vi "ReadSensorValues_v1.1.vi"(1 "Sample time reference sensor / s":dbl=1.0, 2 "VISA resource name":refnum<visa-resource-name>, 3 "Sensor type":T1) -> ()   [LabVIEW 2012]
uses:
  <vilib>/nican/nicantsk.llb/CAN Interface.ctl
  SensorTypes.ctl
  SensorStates.ctl
  <vilib>/nican/nicantsk.llb/CAN Task Reference.ctl
  <vilib>/nican/nicantsk.llb/CAN Mode.ctl
  globalVariables.vi
  <vilib>/nican/nicantsk.llb/CAN Read Multi Chan Single Samp 1D Dbl.vi
  <instrlib>/Agilent 34970/Agilent 34970.lvlib
panel:
  in  "VISA resource name 2":refnum<visa-resource-name>="USB0::0x0957::0x2007::MY49004365::INSTR"
  in  "Cancel Measurement":bool
  out "new data":bool
  out "running":bool
  out "Sample number":i32
  in  "CAN Interface":T2 items=["CAN0"=0, "CAN1"=1, "CAN2"=2, "CAN3"=3, "CAN4"=4, "CAN5"=5, "CAN6"=6, "CAN7"=7, "CAN8"=8, "CAN9"=9, "CAN10"=10, "CAN11"=11, "CAN12"=12, "CAN13"=13, "CAN14"=14, "CAN15"=15, "CAN16"=16, "CAN17"=17, "CAN18"=18, "CAN19"=19, "CAN20"=20, "CAN21"=21, "CAN22"=22, "CAN23"=23, "CAN24"=24, "CAN25"=25, "CAN26"=26, "CAN27"=27, "CAN28"=28, "CAN29"=29, "CAN30"=30, "CAN31"=31, "CAN32"=32, "CAN33"=33, "CAN34"=34, "CAN35"=35, "CAN36"=36, "CAN37"=37, "CAN38"=38, "CAN39"=39, "CAN40"=40, "CAN41"=41, "CAN42"=42, "CAN43"=43, "CAN44"=44, "CAN45"=45, "CAN46"=46, "CAN47"=47, "CAN48"=48, "CAN49"=49, "CAN50"=50, "CAN51"=51, "CAN52"=52, "CAN53"=53, "CAN54"=54, "CAN55"=55, "CAN56"=56, "CAN57"=57, "CAN58"=58, "CAN59"=59, "CAN60"=60, "CAN61"=61, "CAN62"=62, "CAN63"=63, "MAX default"=64, "CAN256 (Virtual)"=256, "CAN257 (Virtual)"=257]
  out "Error Flag":bool
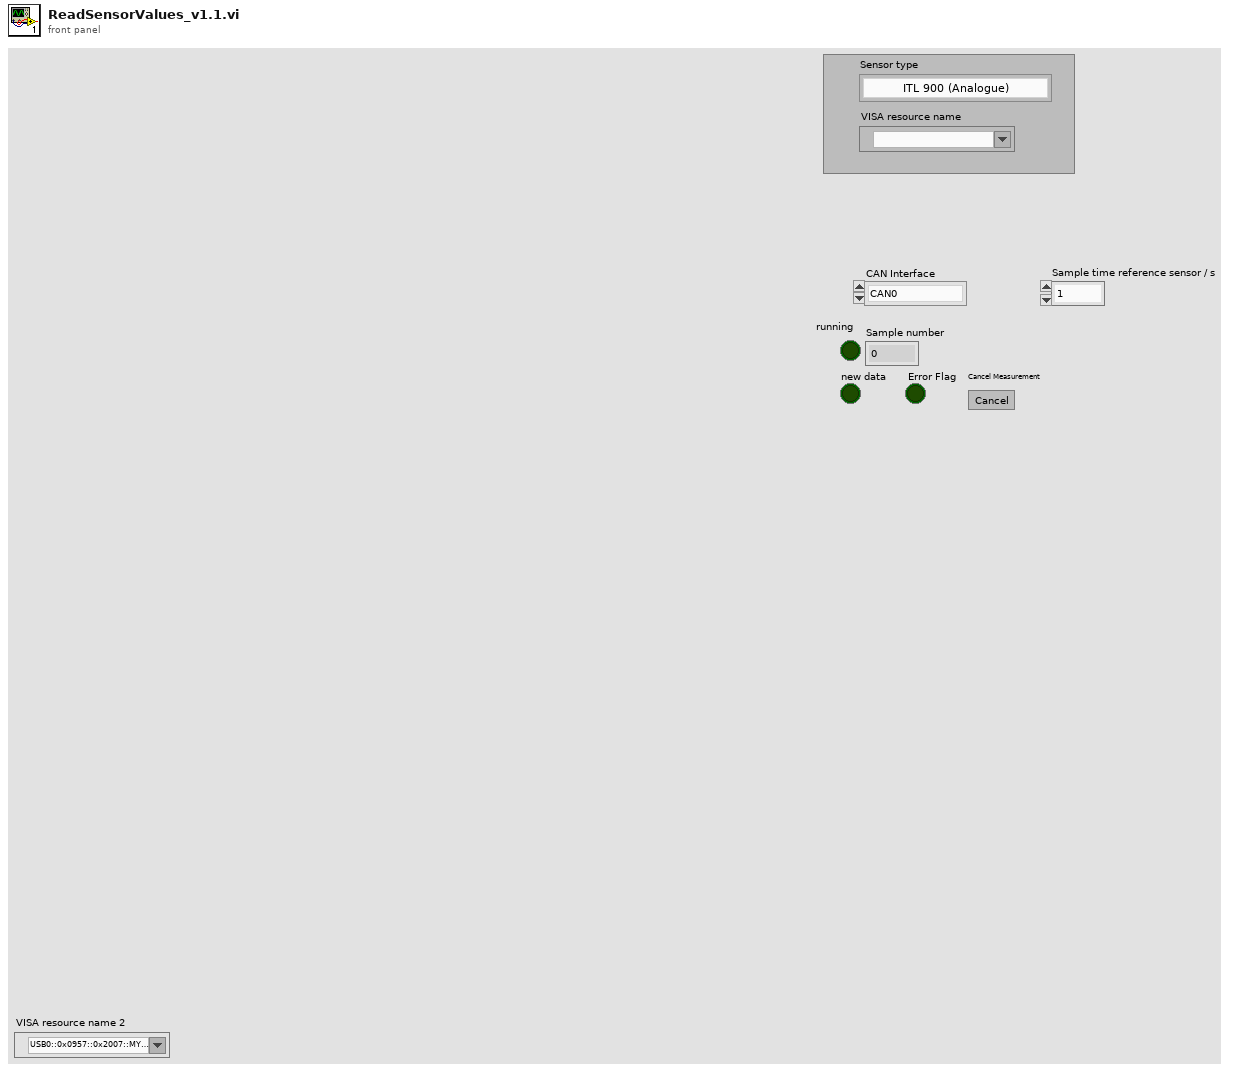
[diagram p1: front panel]
types:
  T1 = typedef "SensorTypes.ctl" = enum16{"ITL 900 (Analogue)", "CAB 300-C SP3 (CAN)", "xyz TODO (PWM)", "xyz TODO (LIN)", "xyz TODO (Analogue)"}
  T2 = typedef "CAN Interface.ctl" = u16
  T3 = typedef "SensorStates.ctl" = enum16{"init", "measure", "terminate"}
  T4 = cluster{"Include Alarm Data F:(No)":bool, "Include Channel # (F:No)":bool, "Include Time (F:No)":bool, "Include Units (F:No)":bool}
  T5 = cluster{"Aperture Value (.4)":dbl, "Aperture (1:Minimum)":u16, "NPLC (1)":u16, "Bandwidth (3 Hz)":u16, "Input Impedance (F:Fixed)":bool, "Integration Time (F:Aperture)":bool}
  T6 = enum16{"100 mV", "1 V", "10 V", "100 V", "300 V", "Minimum", "Maximum"}
  T7 = enum16{"Manual", "Minimum", "Maximum", "Infinity"}
  T8 = enum16{"Bus", "Immediate", "External", "Alarm 1", "Alarm 2", "Alarm 3", "Alarm 4", "Timer"}
  T9 = cluster{"Timeout Value (10000)":u32, "Baud Rate (57600)":enum16{"1200", "2400", "4800", "9600", "19200", "38400", "57600", "115200"}, "Flow Control (1:XON/XOFF)":enum16{"None", "XON / XOFF", "RTS / CTS", "DTR / DSR"}}
  T10 = typedef "CAN Task Reference.ctl" = u32
  T11 = enum16{"Remote Trigger", "Immediate Trigger", "Wait for Trigger", "Abort Scan"}
  T12 = typedef "CAN Mode.ctl" = u16
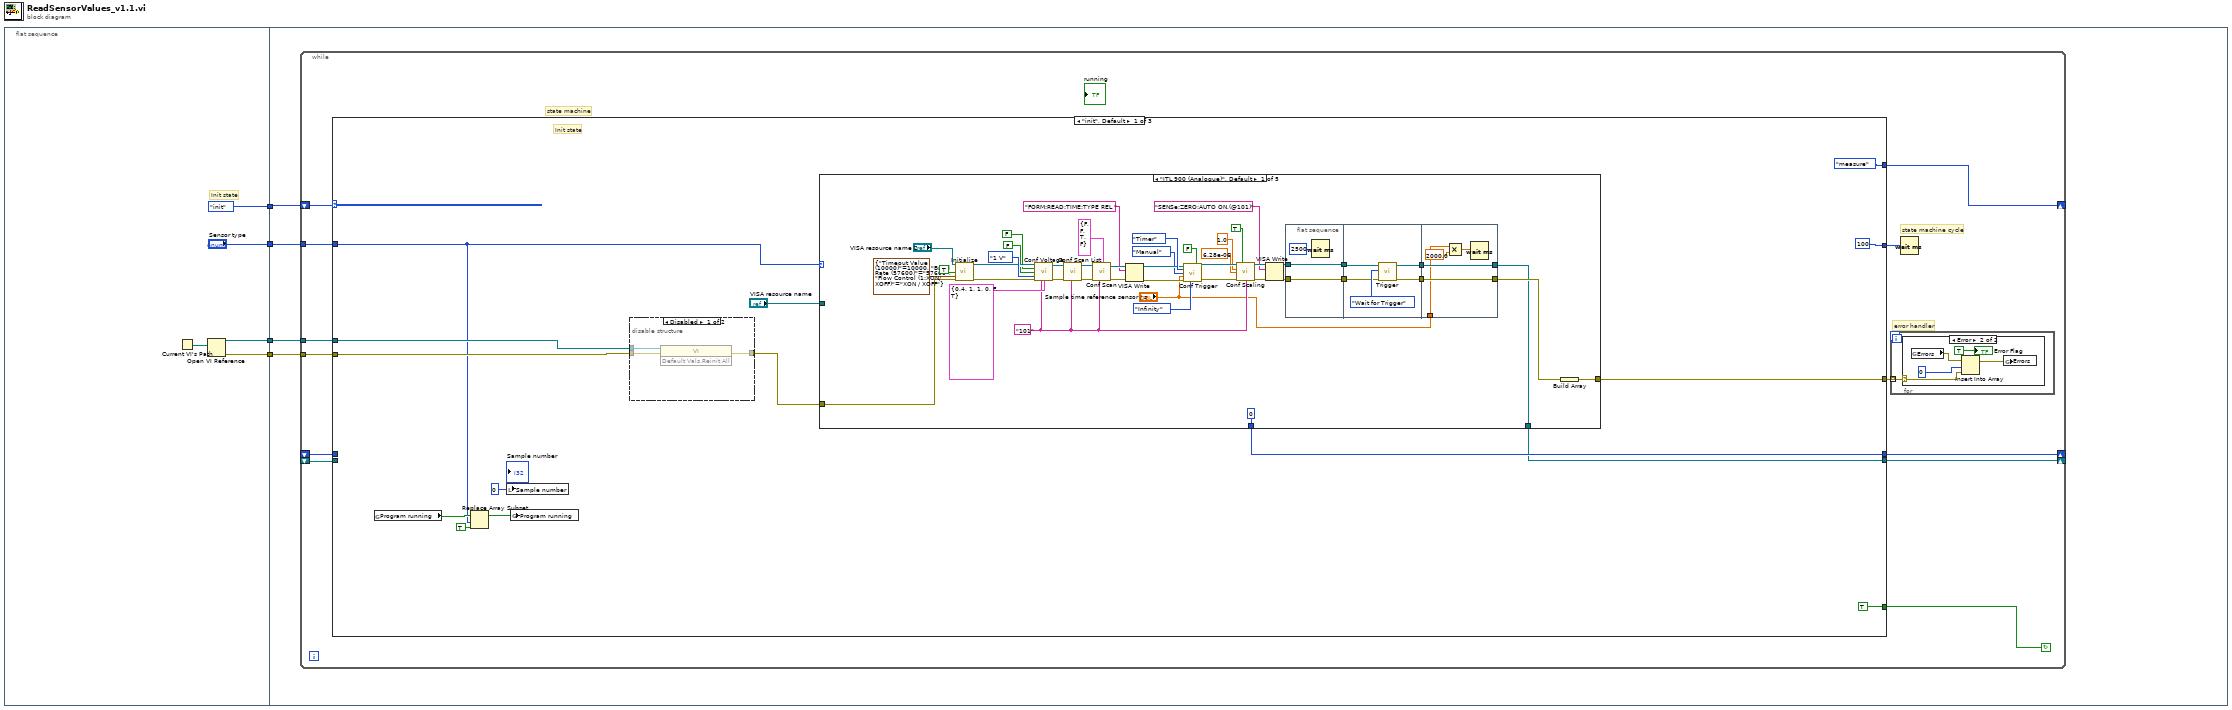
[diagram p0: block diagram]
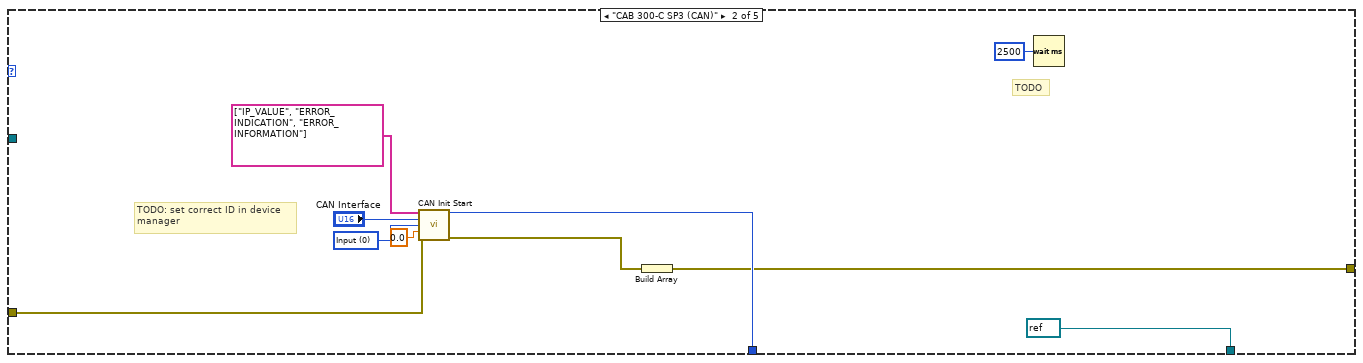
[diagram p4: hidden frame]
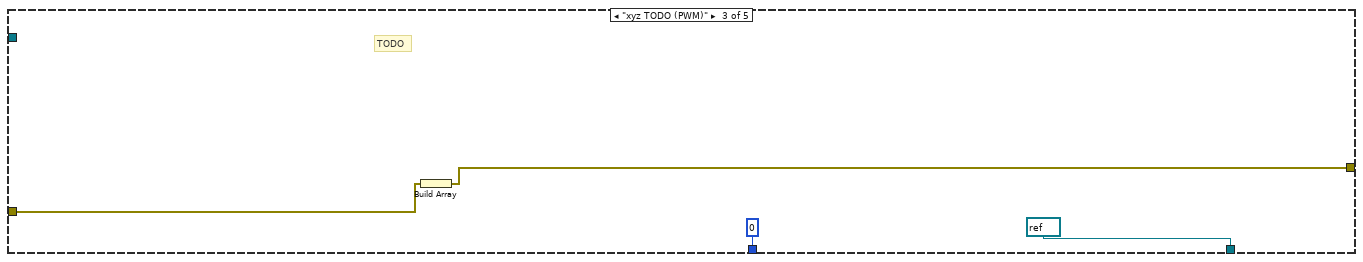
[diagram p5: hidden frame]
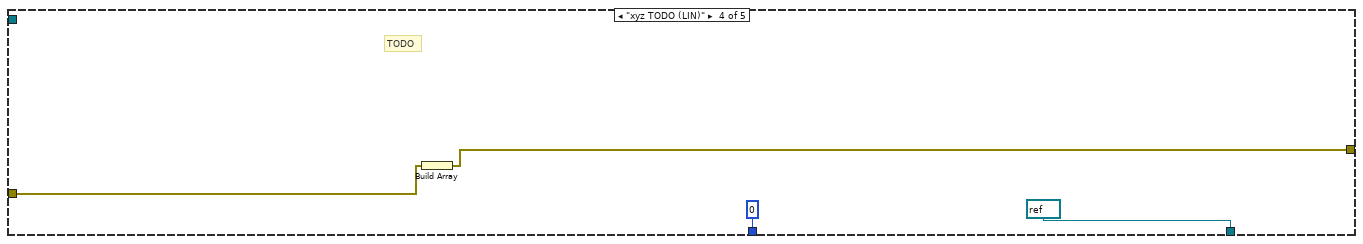
[diagram p6: hidden frame]
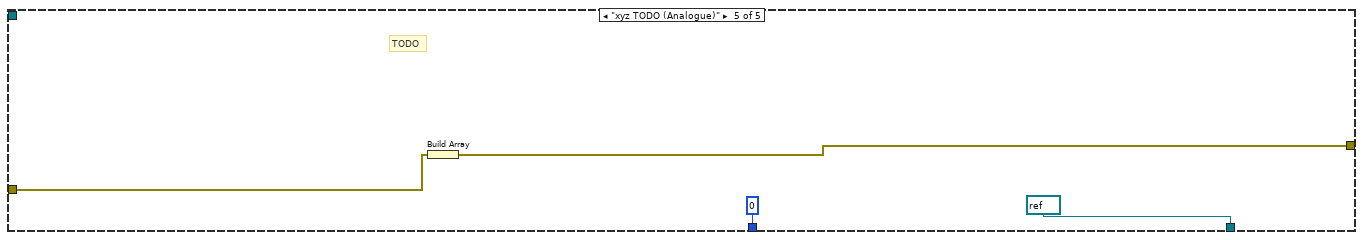
[diagram p7: hidden frame]
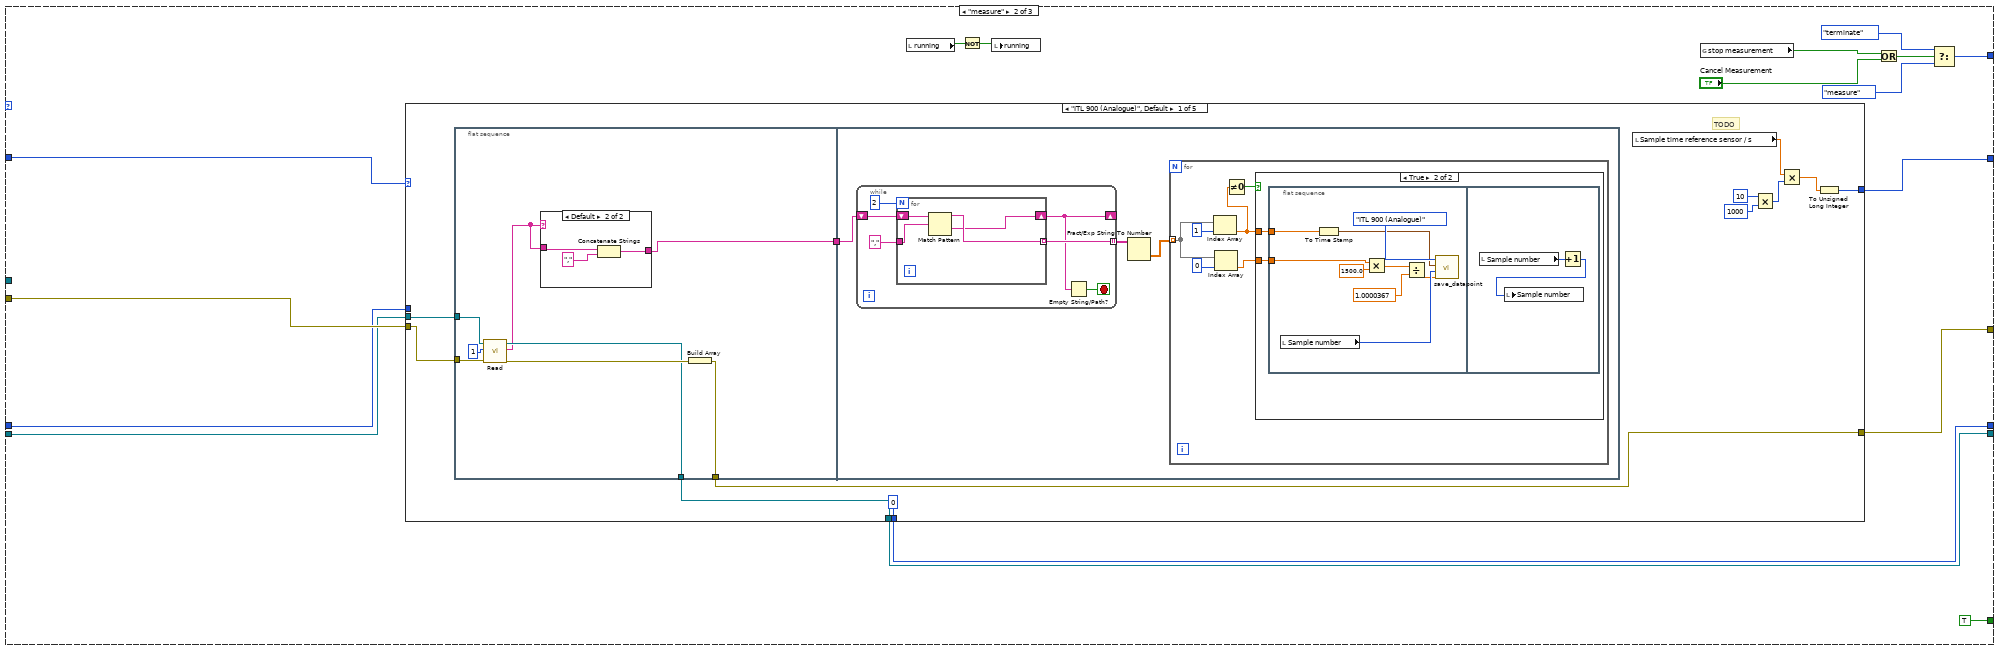
[diagram p8: hidden frame]
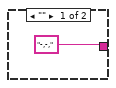
[diagram p9: hidden frame]
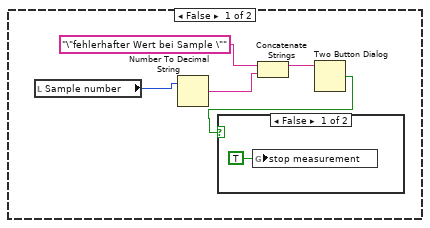
[diagram p10: hidden frame]
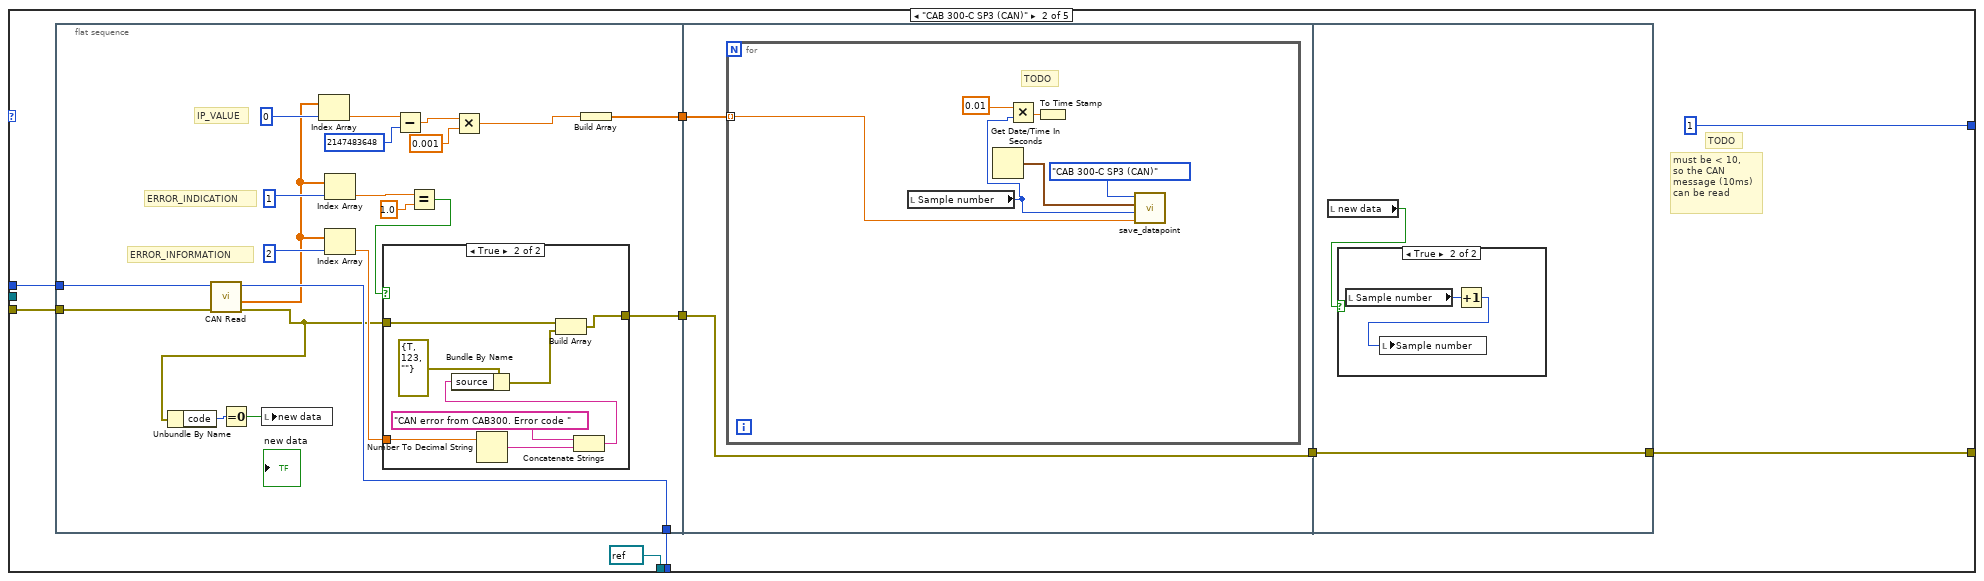
[diagram p12: hidden frame]
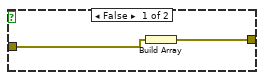
[diagram p13: hidden frame]
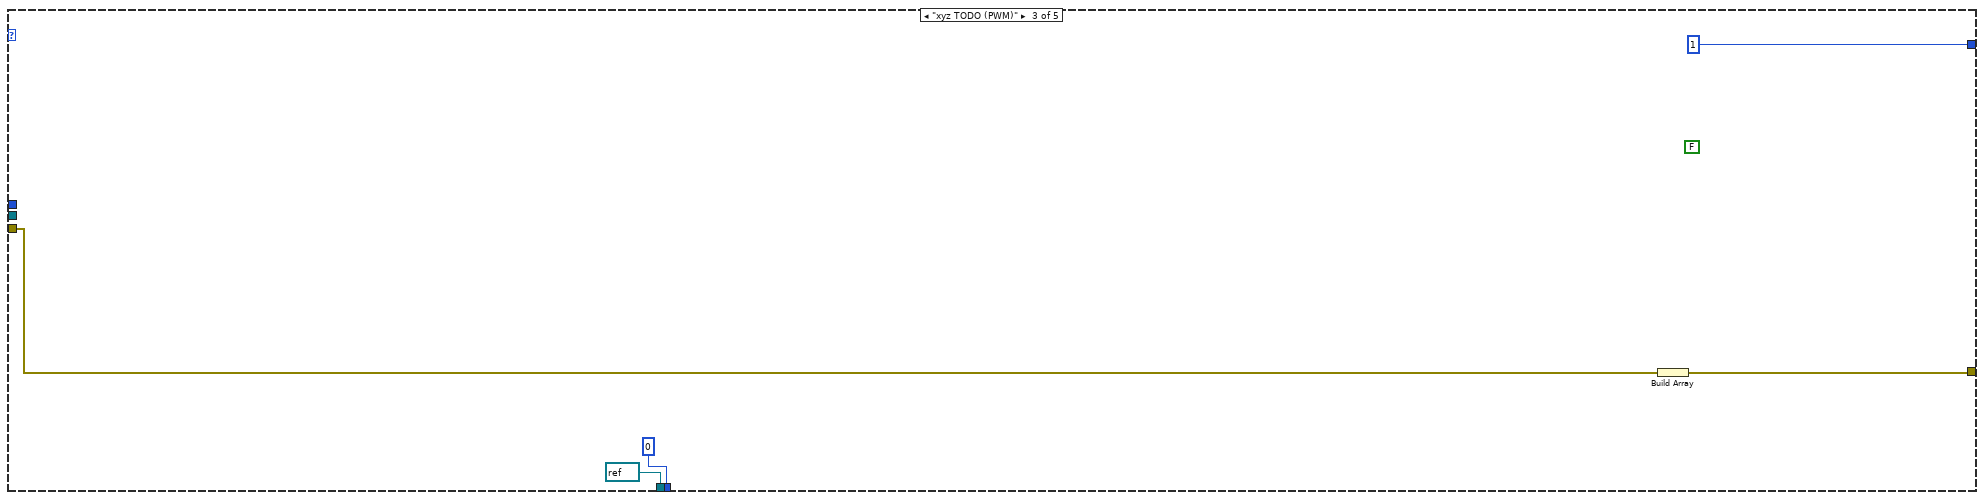
[diagram p15: hidden frame]
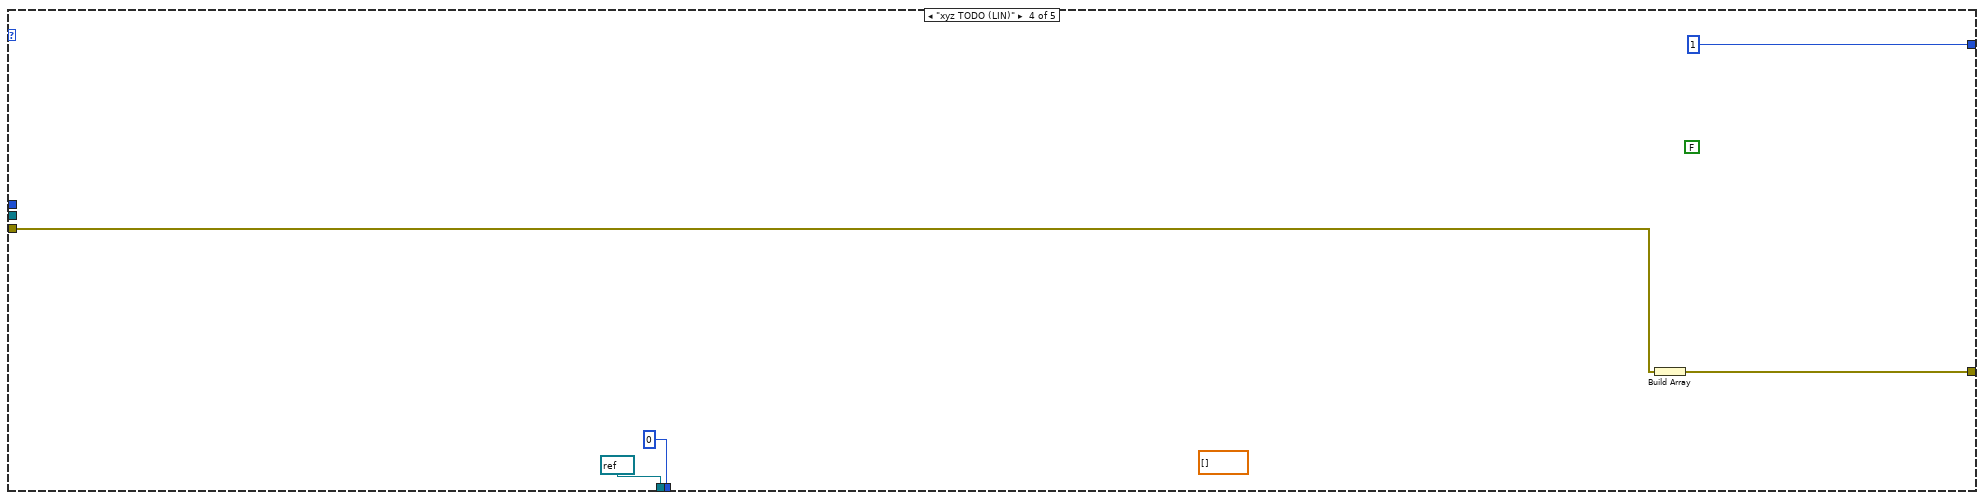
[diagram p16: hidden frame]
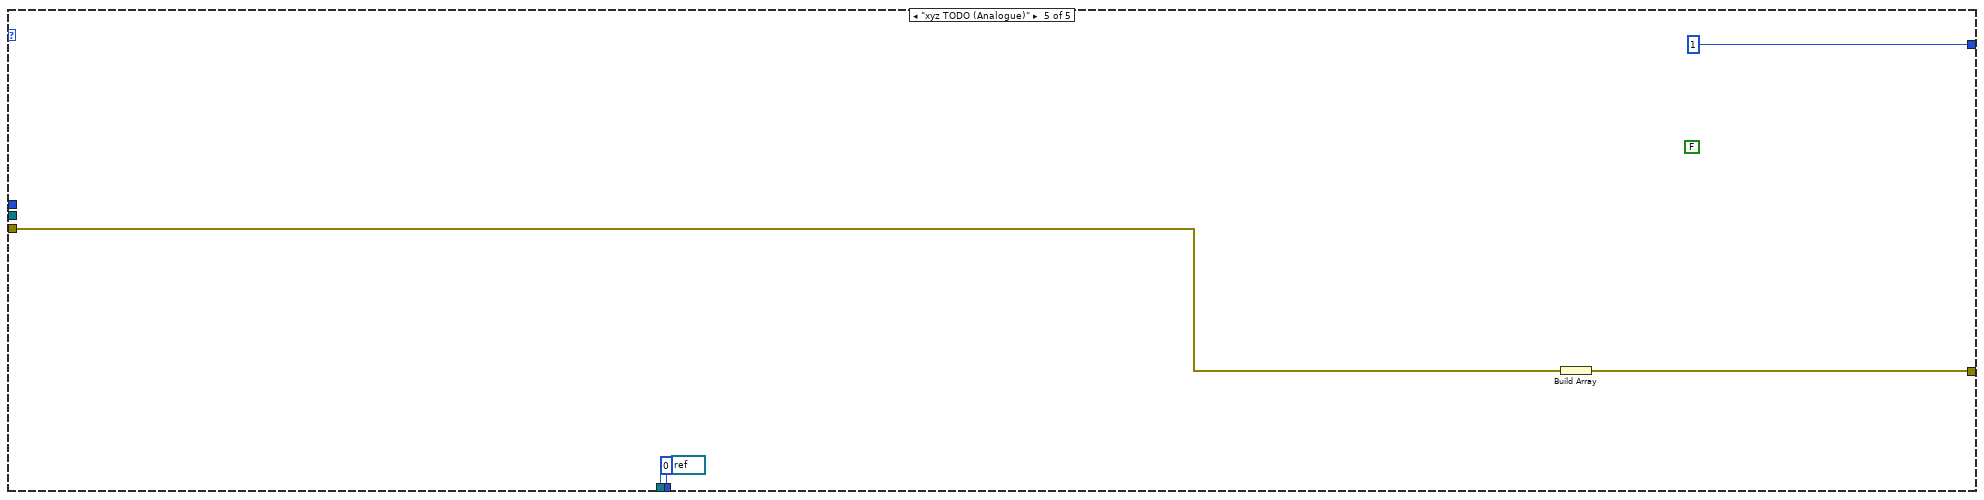
[diagram p17: hidden frame]
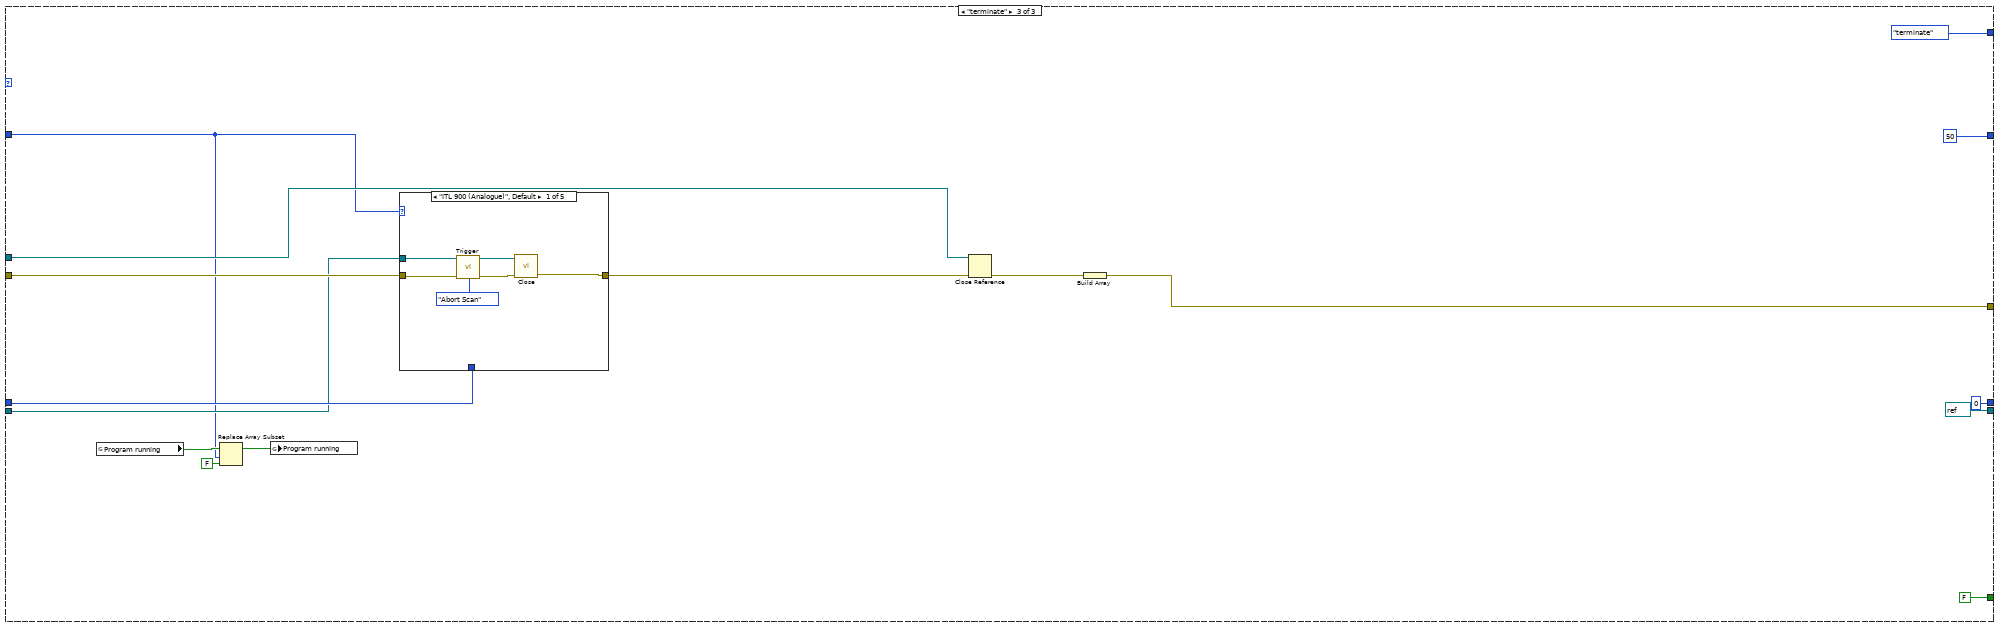
[diagram p18: hidden frame]
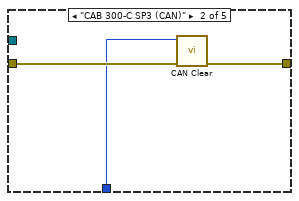
[diagram p19: hidden frame]
diagram:
  n1 = flat-sequence {
    tunnel: [SensorStates."init" ("States IEEE-488")] -> w4
    tunnel: [w9] -> w3
    tunnel: [w8] -> w2
    tunnel: ["Sensor type"] -> w1
    tunnel: w4 -> [w11]
    tunnel: w3 -> [w13]
    tunnel: w2 -> [w12]
    tunnel: w1 -> [w10]
    frame #0 {
      # "Init state"
      n2 = Current VI's Path() -> (path=w7:path)
      n3 = Open VI Reference(vi path=w7) -> (vi reference=w9:refnum<vi>, error out=w8:errorcluster)  [unwired: 2 in, 3 out]
    }
    frame #1 {
      n4 = while {
        tunnel: w13 -> [w24]
        tunnel: w12 -> [w23]
        shift-right: [w21] -> _
        shift-left: w11 -> [w22]
        shift-right: [w20] -> _
        shift-left: _ -> [w19]
        tunnel: w10 -> [w17]
        shift-right: [w16] -> _
        shift-left: _ -> [w15]
        stop <- w14 continue-if-true
        # "state machine"
        # "error handler"
        # "state machine cycle"
        n5 = case shown="\"init\", Default" w22 {
          tunnel: [u32 100 ("milliseconds to wait") w129 u32 50 ("milliseconds to wait")] -> w25
          tunnel: w24 -> [w44 _ w283]
          tunnel: w23 -> [w45 w142 w287]
          tunnel: [SensorStates."measure" ("States IEEE-488") w143 SensorStates."terminate" ("States IEEE-488")] -> w21
          tunnel: [w42 w136 T10 0 ("task reference out")] -> w20
          tunnel: w19 -> [_ w137 w286]
          tunnel: [w40 w138 w285] -> w18
          tunnel: w17 -> [w32 w130 w275]
          tunnel: [TRUE TRUE FALSE] -> w14
          tunnel: [w36 w131 refnum<visa-resource-name> refnum ("VISA Resource Name Out")] -> w16
          tunnel: w15 -> [_ w132 w280]
          frame "init", Default {
            # "Init state"
            n6 = global read "globalVariables.vi" "Program running"() -> (w35:bool[])
            n7 = Replace Array Subset(array=w35, new element=TRUE ("new element/subarray"), index=w32) -> (w34:bool[])
            n8 = local write "Sample number"(0 ("Sample number")) -> ()
            n9 = global write "globalVariables.vi" "Program running"(w34) -> ()
            n10 = disable-structure shown="Disabled" {
              disable-tunnel: w45 -> [w49 _]
              disable-tunnel: w44 -> [w48 _]
              disable-tunnel: [w47 _] -> w41
              frame Disabled {
                n11 = invoke class="VI" method="Default Vals.Reinit All"(reference=w48, error in=w49) -> (error out=w47:errorcluster)  [unwired: 1 in, 2 out]
              }
              frame Enabled {
              }
            }
            n12 = case shown="\"ITL 900 (Analogue)\", Default" w32 {
              tunnel: [T10 0 ("task reference out") w112 T10 0 ("task reference out") T10 0 ("task reference out") T10 0 ("task reference out")] -> w42
              tunnel: w41 -> [w56 w111 w119 w123 w128]
              tunnel: [w93 w109 w120 w124 w127] -> w40
              tunnel: "VISA resource name" -> [_ _ _ _ _]
              tunnel: [w54 refnum<visa-resource-name> refnum ("VISA Resource Name Out") refnum<visa-resource-name> refnum ("VISA Resource Name Out") refnum<visa-resource-name> refnum ("VISA Resource Name Out") refnum<visa-resource-name> refnum ("VISA Resource Name Out")] -> w36
              frame "ITL 900 (Analogue)", Default {
                w62 = "101" ("Channel List (Volt.)")
                n13 = call <instrlib>:"Initialize.vi"("VISA Resource Name"="VISA resource name 2", "Reset (T: Reset)"=TRUE, "Serial Port Configuration"=T9 {"Timeout Value (10000)"=10000, "Baud Rate (57600)"=enum."57600", "Flow Control (1:XON/XOFF)"=enum."XON / XOFF"}, "error in (no error)"=w56) -> ("VISA Resource Name Out"=w87:refnum<visa-resource-name>, "error out"=w83:errorcluster)  [unwired: 10 in]
                n14 = call <instrlib>:"Conf Voltage.vi"("VISA Resource Name"=w87, "AC/DC (F:DC)"=FALSE, "Autorange? (F:Off)"=FALSE, "Range (6:Max)"=T6."1 V" ("Range (Volt.)"), "error in (no error)"=w83, "Channel List (empty)"=w62, "Advanced Config"=T5 {"Aperture Value (.4)"=0.4, "Aperture (1:Minimum)"=1, "NPLC (1)"=1, "Bandwidth (3 Hz)"=0, "Input Impedance (F:Fixed)"=FALSE, "Integration Time (F:Aperture)"=TRUE}) -> ("VISA Resource Name Out"=w85:refnum<visa-resource-name>, "error out"=w80:errorcluster)  [unwired: 6 in, 1 out]
                n15 = call <instrlib>:"Conf Scan List.vi"("Scan List (empty)"=w62, "error in (no error)"=w80, "VISA Resource Name"=w85) -> ("error out"=w79:errorcluster, "VISA Resource Name Out"=w81:refnum<visa-resource-name>)  [unwired: 6 in, 1 out]
                n16 = call <instrlib>:"Conf Scan.vi"("VISA Resource Name"=w81, "error in (no error)"=w79, "Channel List (empty)"=w62, "Scan Fields"=T4 {"Include Alarm Data F:(No)"=FALSE, "Include Channel # (F:No)"=FALSE, "Include Time (F:No)"=TRUE, "Include Units (F:No)"=FALSE}) -> ("VISA Resource Name Out"=w75:refnum<visa-resource-name>, "error out"=w74:errorcluster)  [unwired: 9 in, 1 out]
                n17 = VISA Write(VISA resource name=w75, write buffer="FORM:READ:TIME:TYPE REL ", error in (no error)=w74) -> (VISA resource name out=w72:refnum<visa-resource-name>, error out=w73:errorcluster)  [unwired: 1 out]
                n18 = call <instrlib>:"Conf Trigger.vi"("VISA Resource Name"=w72, "Wait for Trigger? (F:No)"=FALSE, "Source (1:Immediate)"=T8."Timer", "Time-Scan Interval (1:Min)"=enum16{"Manual", "Minimum", "Maximum"}."Manual", "Interval Value (0)"="Sample time reference sensor / s", "error in (no error)"=w73, "Max Trigger Count (3:Inf)"=T7."Infinity") -> ("VISA Resource Name Out"=w66:refnum<visa-resource-name>, "error out"=w65:errorcluster)  [unwired: 6 in, 1 out]
                n19 = call <instrlib>:"Conf Scaling.vi"("VISA Resource Name"=w66, "Enable Scaling? (T:Enable)"=TRUE, "Gain (1)"=1.0, "Offset (0)"=6.28e-06, "error in (no error)"=w65, "Channel List (empty)"=w62) -> ("VISA Resource Name Out"=w61:refnum<visa-resource-name>, "error out"=w60:errorcluster)  [unwired: 7 in, 1 out]
                n20 = VISA Write(VISA resource name=w61, write buffer="SENSe:ZERO:AUTO ON,(@101)", error in (no error)=w60) -> (VISA resource name out=w59:refnum<visa-resource-name>, error out=w58:errorcluster)  [unwired: 1 out]
                n21 = flat-sequence {
                  tunnel: [w95] -> w91
                  tunnel: w59 -> [w95]
                  tunnel: [w94] -> w90
                  tunnel: w58 -> [w94]
                  tunnel: w91 -> [w98]
                  tunnel: w90 -> [w97]
                  tunnel: [w101] -> w52
                  tunnel: [w100] -> w51
                  tunnel: [w105] -> w55
                  tunnel: [w106] -> w54
                  tunnel: w52 -> [w106]
                  tunnel: w51 -> [w105]
                  tunnel: "Sample time reference sensor / s" -> [w103]
                  frame #0 {
                    n22 = Wait (ms)(milliseconds to wait=u32 2500) -> ()  [unwired: 1 out]
                  }
                  frame #1 {
                    n23 = call <instrlib>:"Trigger.vi"("error in (no error)"=w97, "Command (0:Rem Trig)"=T11."Wait for Trigger", "VISA Resource Name"=w98) -> ("error out"=w100:errorcluster, "VISA Resource Name Out"=w101:refnum<visa-resource-name>)  [unwired: 7 in]
                  }
                  frame #2 {
                    n24 = Multiply(x=w103, y=2000.0) -> (x*y=w104:dbl)
                    n25 = Wait (ms)(milliseconds to wait=w104) -> ()  [unwired: 1 out]
                  }
                }
                n26 = Build Array(w55) -> (w93:errorcluster[])
              }
              frame "CAB 300-C SP3 (CAN)" {
                w113 = T12 0 items=["Input", "Output", "Timestamped Input", "Output Recent"] ("mode")
                # "TODO"
                # "TODO: set correct ID in device\nmanager"
                n27 = call <vilib>:"CAN Init Start.vi"("channel list"=string[] ["IP_VALUE", "ERROR_INDICATION", "ERROR_INFORMATION"] ("Channel List"), "interface"="CAN Interface", "mode"=w113, "sample rate"=0.0, "error in (no error)"=w111) -> ("task reference out"=w112:T10, "error out"=w110:errorcluster)  [unwired: 9 in]
                n28 = Build Array(w110) -> (w109:errorcluster[])
                n29 = Wait (ms)(milliseconds to wait=u32 2500) -> ()  [unwired: 1 out]
              }
              frame "xyz TODO (PWM)" {
                # "TODO"
                n30 = Build Array(w119) -> (w120:errorcluster[])
              }
              frame "xyz TODO (LIN)" {
                # "TODO"
                n31 = Build Array(w123) -> (w124:errorcluster[])
              }
              frame "xyz TODO (Analogue)" {
                # "TODO"
                n32 = Build Array(w128) -> (w127:errorcluster[])
              }
            }
          }
          frame "measure" {
            n33 = case shown="\"ITL 900 (Analogue)\", Default" w130 {
              tunnel: w142 -> [w156 w213 w263 w267 w272]
              tunnel: [w153 w212 w264 w268 w273] -> w138
              tunnel: w137 -> [_ w211 _ _ _]
              tunnel: [T10 0 ("task reference out") w210 T10 0 ("task reference out") T10 0 ("task reference out") T10 0 ("task reference out")] -> w136
              tunnel: w132 -> [w157 _ _ _ _]
              tunnel: [w154 refnum<visa-resource-name> refnum ("VISA Resource Name Out") refnum<visa-resource-name> refnum ("VISA Resource Name Out") refnum<visa-resource-name> refnum ("VISA Resource Name Out") refnum<visa-resource-name> refnum ("VISA Resource Name Out")] -> w131
              tunnel: [w147 u32 1 ("milliseconds to wait") u32 1 ("milliseconds to wait") u32 1 ("milliseconds to wait") u32 1 ("milliseconds to wait")] -> w129
              frame "ITL 900 (Analogue)", Default {
                # "TODO"
                n34 = flat-sequence {
                  tunnel: w157 -> [w163]
                  tunnel: w156 -> [w162]
                  tunnel: [w161] -> w155
                  tunnel: [w160] -> w154
                  tunnel: [w159] -> w153
                  tunnel: w155 -> [w172]
                  frame #0 {
                    n35 = call <instrlib>:"Read.vi"("error in (no error)"=w162, "# Channels (1)"=1, "VISA Resource Name"=w163) -> ("error out"=w164:errorcluster, "Readings"=w158:string, "VISA Resource Name Out"=w160:refnum<visa-resource-name>)  [unwired: 5 in, 1 out]
                    n36 = case shown="Default" w158 {
                      tunnel: ["-,-," ("string") w169] -> w161
                      tunnel: w158 -> [_ w168]
                      frame "" {
                      }
                      frame Default {
                        n37 = Concatenate Strings(w168, "," ("string")) -> (w169:string)
                      }
                    }
                    n38 = Build Array(w164) -> (w159:errorcluster[])
                  }
                  frame #1 {
                    n39 = while {
                      tunnel: [w177] -> w171 mode=indexing
                      shift-left: w172 -> [w178]
                      shift-right: [w174] -> _
                      stop <- w176 stop-if-true
                      n40 = for {
                        N: 2 -> [_]
                        tunnel: [w180] -> w177 mode=indexing
                        tunnel: "," ("regular expression") -> [w181]
                        shift-right: [w179] -> w174
                        shift-left: w178 -> [w182]
                        n41 = Match Pattern(string=w182, regular expression=w181) -> (before substring=w180:string, after substring=w179:string)  [unwired: 1 in, 2 out]
                      }
                      n42 = Empty String/Path?(string/path=w174) -> (empty?=w176:bool)
                    }
                    n43 = Fract/Exp String To Number(string=w171) -> (number=w170:dbl[][])  [unwired: 3 in, 1 out]
                    n44 = for {
                      tunnel: w170 -> [w186] mode=indexing
                      n45 = Index Array(array=w186, index=1 ("disabled index (col)")) -> (element=w183:dbl)
                      n46 = Index Array(array=w186, index=0 ("disabled index (col)")) -> (element=w185:dbl)
                      n47 = Not Equal To 0?(x=w183) -> (x != 0?=w184:bool)
                      n48 = case shown="True" w184 {
                        tunnel: w183 -> [_ w196]
                        tunnel: w185 -> [_ w195]
                        frame False {
                          n49 = local read "Sample number"() -> (w193:i32)
                          n50 = Number To Decimal String(number=w193) -> (decimal integer string=w190:string)  [unwired: 1 in]
                          n51 = Concatenate Strings("\"fehlerhafter Wert bei Sample \"" ("message"), w190) -> (w192:string)
                          n52 = Two Button Dialog(message=w192) -> (T button?=w189:bool)  [unwired: 2 in]
                          n53 = case shown="False" w189 {
                            frame False {
                              n54 = global write "globalVariables.vi" "stop measurement"(TRUE ("stop measurement")) -> ()
                            }
                            frame True {
                            }
                          }
                        }
                        frame True {
                          n55 = flat-sequence {
                            tunnel: w196 -> [w197]
                            tunnel: w195 -> [w198]
                            frame #0 {
                              n56 = local read "Sample number"() -> (w204:i32)
                              n57 = To Time Stamp(1:w197) -> (0:w199:timestamp)
                              n58 = Multiply(x=w198, y=1500.0) -> (x*y=w201:dbl)
                              n59 = Divide(x=w201, y=1.0000367) -> (x/y=w200:dbl)
                              n60 = call "save_datapoint.vi"("current value"=w200, "Sample number"=w204, "current time of measurement"=w199, "Sensor type"=SensorTypes."ITL 900 (Analogue)") -> ()
                            }
                            frame #1 {
                              n61 = local read "Sample number"() -> (w207:i32)
                              n62 = Increment(x=w207) -> (x+1=w206:i32)
                              n63 = local write "Sample number"(w206) -> ()
                            }
                          }
                        }
                      }
                    }
                  }
                }
                n64 = local read "Sample time reference sensor / s"() -> (w148:dbl)
                n65 = Multiply(x=u32 10, y=u32 1000) -> (x*y=w149:u32)
                n66 = Multiply(x=w148, y=w149) -> (x*y=w146:dbl)
                n67 = To Unsigned Long Integer(number=w146) -> (unsigned 32bit integer=w147:u32)
              }
              frame "CAB 300-C SP3 (CAN)" {
                # "TODO"
                # "must be < 10,\nso the CAN \nmessage (10ms) \ncan be read"
                n68 = flat-sequence {
                  tunnel: [w236] -> w216
                  tunnel: [w235] -> w215
                  tunnel: w213 -> [w237]
                  tunnel: w211 -> [w234]
                  tunnel: [w233] -> w210
                  tunnel: w216 -> [w249]
                  tunnel: w215 -> [w248]
                  tunnel: [w249] -> w214
                  tunnel: w214 -> [w257]
                  tunnel: [w257] -> w212
                  frame #0 {
                    # "ERROR_INFORMATION"
                    # "ERROR_INDICATION"
                    # "IP_VALUE"
                    n69 = call-poly <vilib>:"CAN Read.vi"("error in (no error)"=w237, "task reference in"=w234) -> ("error out"=w224:errorcluster, "multi-chan single-samp 1D dbl"=w227:dbl[], "task reference out"=w233:T10)  [unwired: 6 in, 1 out]
                    n70 = Unbundle By Name(w224) -> ("code"=w223:i32)
                    n71 = Equal To 0?(x=w223) -> (x = 0?=w222:bool)
                    n72 = local write "new data"(w222) -> ()
                    n73 = Index Array(array=w227, index=0) -> (element=w221:dbl)
                    n74 = Index Array(array=w227, index=1) -> (element=w229:dbl)
                    n75 = Index Array(array=w227, index=2) -> (element=w226:dbl)
                    n76 = Subtract(x=w221, y=u32 2147483648) -> (x-y=w219:dbl)
                    n77 = Equal?(x=w229, y=1.0) -> (x = y?=w225:bool)
                    n78 = case shown="True" w225 {
                      tunnel: w224 -> [w239 w247]
                      tunnel: [w238 w246] -> w236
                      tunnel: w226 -> [_ w241]
                      frame False {
                        n79 = Build Array(w239) -> (w238:errorcluster[])
                      }
                      frame True {
                        n80 = Number To Decimal String(number=w241) -> (decimal integer string=w242:string)  [unwired: 1 in]
                        n81 = Concatenate Strings("CAN error from CAB300. Error code ", w242) -> (w240:string)
                        n82 = Bundle By Name(cluster=errorcluster {"status"=TRUE, "code"=123, "source"=""} ("error out"), "source"=w240) -> (w244:errorcluster)
                        n83 = Build Array(w247, w244) -> (w246:errorcluster[])
                      }
                    }
                    n84 = Multiply(x=w219, y=0.001) -> (x*y=w217:dbl)
                    n85 = Build Array(w217) -> (w235:dbl[])
                  }
                  frame #1 {
                    n86 = for {
                      tunnel: w248 -> [w254] mode=indexing
                      # "TODO"
                      n87 = local read "Sample number"() -> (w252:i32)
                      n88 = Get Date/Time In Seconds() -> (seconds since 1Jan1904=w251:timestamp)
                      n89 = Multiply(x=0.01, y=w252) -> (x*y=w250:dbl)
                      n90 = To Time Stamp(1:w250) -> ()  [unwired: 1 out]
                      n91 = call "save_datapoint.vi"("current value"=w254, "Sample number"=w252, "current time of measurement"=w251, "Sensor type"=SensorTypes."CAB 300-C SP3 (CAN)") -> ()
                    }
                  }
                  frame #2 {
                    n92 = local read "new data"() -> (w256:bool)
                    n93 = case shown="True" w256 {
                      frame False {
                      }
                      frame True {
                        n94 = local read "Sample number"() -> (w259:i32)
                        n95 = Increment(x=w259) -> (x+1=w258:i32)
                        n96 = local write "Sample number"(w258) -> ()
                      }
                    }
                  }
                }
              }
              frame "xyz TODO (PWM)" {
                (unwired) FALSE ("new data")
                n97 = Build Array(w263) -> (w264:errorcluster[])
              }
              frame "xyz TODO (LIN)" {
                (unwired) dbl[] []
                (unwired) FALSE ("new data")
                n98 = Build Array(w267) -> (w268:errorcluster[])
              }
              frame "xyz TODO (Analogue)" {
                (unwired) FALSE ("new data")
                n99 = Build Array(w272) -> (w273:errorcluster[])
              }
            }
            n100 = local read "running"() -> (w140:bool)
            n101 = Not(x=w140) -> (.not. x?=w141:bool)
            n102 = local write "running"(w141) -> ()
            n103 = global read "globalVariables.vi" "stop measurement"() -> (w135:bool)
            n104 = Or(x=w135, y="Cancel Measurement") -> (x .or. y?=w133:bool)
            n105 = Select(t=SensorStates."terminate" ("States IEEE-488"), s=w133, f=SensorStates."measure" ("States IEEE-488")) -> (s? t:f=w143:T3)
          }
          frame "terminate" {
            n106 = global read "globalVariables.vi" "Program running"() -> (w278:bool[])
            n107 = Replace Array Subset(array=w278, new element=FALSE ("new element/subarray"), index=w275) -> (w277:bool[])
            n108 = global write "globalVariables.vi" "Program running"(w277) -> ()
            n109 = case shown="\"ITL 900 (Analogue)\", Default" w275 {
              tunnel: w287 -> [w293 w299 w300 w301 w302]
              tunnel: [w292 w298 w300 w301 w302] -> w282
              tunnel: w286 -> [_ w297 _ _ _]
              tunnel: w280 -> [w291 _ _ _ _]
              frame "ITL 900 (Analogue)", Default {
                n110 = call <instrlib>:"Trigger.vi"("error in (no error)"=w293, "Command (0:Rem Trig)"=T11."Abort Scan", "VISA Resource Name"=w291) -> ("error out"=w295:errorcluster, "VISA Resource Name Out"=w294:refnum<visa-resource-name>)  [unwired: 7 in]
                n111 = call <instrlib>:"Close.vi"("VISA Resource Name"=w294, "error in (no error)"=w295) -> ("error out"=w292:errorcluster)  [unwired: 13 in]
              }
              frame "CAB 300-C SP3 (CAN)" {
                n112 = call <vilib>:"CAN Clear.vi"("error in (no error)"=w299, "task reference in"=w297) -> ("error out"=w298:errorcluster)  [unwired: 9 in]
              }
              frame "xyz TODO (PWM)" {
              }
              frame "xyz TODO (LIN)" {
              }
              frame "xyz TODO (Analogue)" {
              }
            }
            n113 = Close Reference(reference=w283, error in (no error)=w282) -> (error out=w289:errorcluster)
            n114 = Build Array(w289) -> (w285:errorcluster[])
          }
        }
        n115 = for {
          tunnel: w18 -> [w26] mode=indexing
          n116 = case shown="Error" w26 {
            selector: w26 -> [_ w30]
            frame No Error {
            }
            frame Error {
              n117 = global read "globalVariables.vi" "Errors"() -> (w28:errorcluster[])
              n118 = Insert Into Array(array=w28, index=0, new element=w30) -> (w27:errorcluster[])
              n119 = global write "globalVariables.vi" "Errors"(w27) -> ()
              "Error Flag" <- TRUE ("Error Flag")
            }
          }
        }
        n120 = Wait (ms)(milliseconds to wait=w25) -> ()  [unwired: 1 out]
      }
    }
  }
